vi "cblas daxpy.vi"(5 "n":i32=-1, 6 "incy":i32=1, 7 "incx":i32=1, 9 "alpha":dbl=1.0, 10 "y":dbl[](array[numeric]), 11 "x":dbl[](array[numeric])) -> (0 "error":i32, 3 "daxpy":dbl[](array[numeric]))   [LabVIEW 2017, in "NI_AALBLAS.lvlib"]
uses:
  NI_AALBLAS.lvlib
  lvblas.dll
panel:
  # "void cblas_daxpy(n, alpha, *x, incx, *y, incy)"
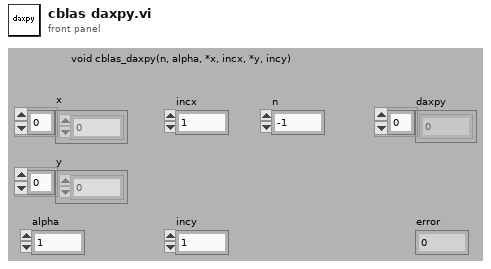
[diagram p1: front panel]
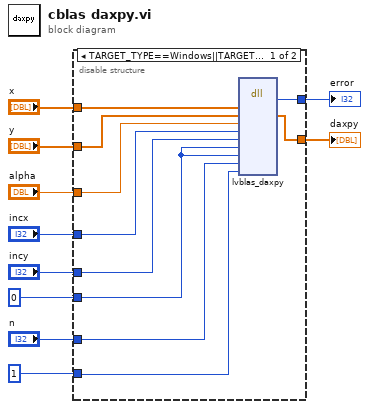
[diagram p0: block diagram]
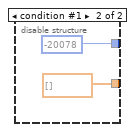
[diagram p2: hidden frame]
diagram:
  n1 = disable-structure shown="TARGET_TYPE==Windows||TARGET_TYPE==Unix||TARGET_TYPE==RT||TARGET_TYPE==Mac" {
    disable-tunnel: "x" -> [w20 _]
    disable-tunnel: "y" -> [w19 _]
    disable-tunnel: [w18 -20078] -> w10
    disable-tunnel: "alpha" -> [w17 _]
    disable-tunnel: "n" -> [w16 _]
    disable-tunnel: [w15 dbl[] []] -> w5
    disable-tunnel: "incx" -> [w14 _]
    disable-tunnel: "incy" -> [w13 _]
    disable-tunnel: 0 -> [w12 _]
    disable-tunnel: 1 -> [w11 _]
    frame condition #0 (active) {
      n2 = dll-call lib="C:/Program Files/National Instruments/LabVIEW 2017/resource/lvblas.*" fn="lvblas_daxpy" ("CBLAS.dll:DotProdH")("X"=w20, "Y"=w19, "alpha"=w17, "IncX"=w14, "IncY"=w13, "startX"=w12, "startY"=w12, "N"=w16, "check"=w11) -> ("error"=w18:i32, "Y"=w15:dbl[])  [unwired: 11 in, 2 out]
    }
    frame condition #1 {
    }
  }
  "daxpy" <- w5
  "error" <- w10
